vi "Deserialize_To_LessSpecific.vi"(8 "error in (no error)":errorcluster, 9 "Error on less-specific wired types?":bool, 10 "To Object":refnum<class>, 11 "From Object":refnum<class>) -> (0 "error out":errorcluster, 3 "Target Object":refnum<class>)   [LabVIEW 2019, in "BlueSerialization.lvlib" / "BlueSerializer.lvclass"]
uses:
  BlueSerializer.lvclass
  <vilib>/ErrorRing/Error Ring.xnode
  <vilib>/Utility/error.llb/Error Cluster From Error Code.vi
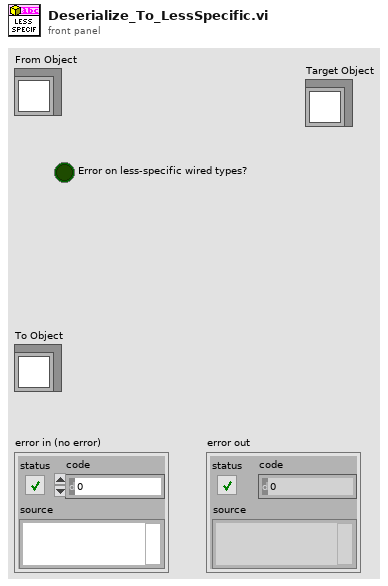
[diagram p1: front panel]
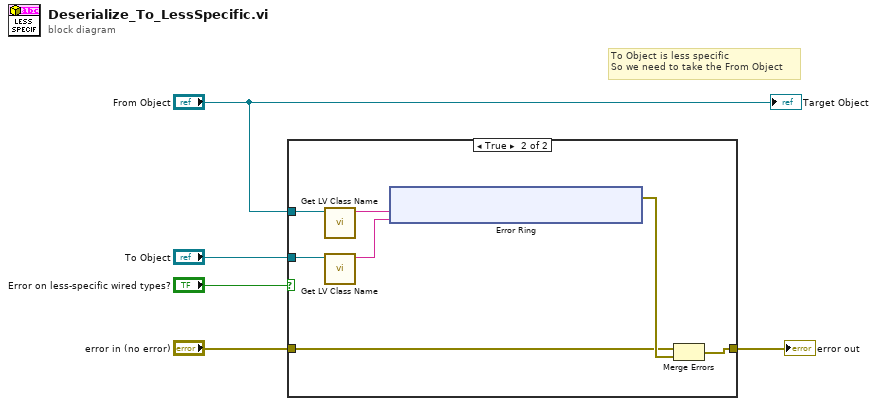
[diagram p0: block diagram]
diagram:
  # "To Object is less specific\nSo we need to take the From Object"
  n1 = case shown="True" "Error on less-specific wired types?" {
    tunnel: "To Object" -> [_ w13]
    tunnel: "From Object" -> [_ w12]
    tunnel: "error in (no error)" -> [w6 w8]
    tunnel: [w6 w7] -> w1
    frame False {
    }
    frame True {
      n2 = call <vilib>:"Get LV Class Name.vi"("object"=w12) -> ("class name"=w11:string)  [unwired: 9 in, 1 out]
      n3 = call <vilib>:"Get LV Class Name.vi"("object"=w13) -> ("class name"=w10:string)  [unwired: 9 in, 1 out]
      n4 = xnode "Error Ring"("parameter 0"=w11, "parameter 1"=w10) -> ("error out"=w9:errorcluster)
      n5 = Merge Errors(w8, w9) -> (w7:errorcluster)
    }
  }
  "error out" <- w1
  "Target Object" <- "From Object"
